vi "串口指令.vi"(7 "write buffer":string, 8 "error in":errorcluster, 9 "是否握手":bool=TRUE, 10 "limit":i32=200, 11 "VISA resource name":refnum<visa-resource-name>) -> (0 "error out":errorcluster, 1 "read buffer ALL":string, 2 "outputString":string, 3 "VISA resource name OUT":refnum<visa-resource-name>, 5 "read buffer HANDSHAKE":string)   [LabVIEW 2016]
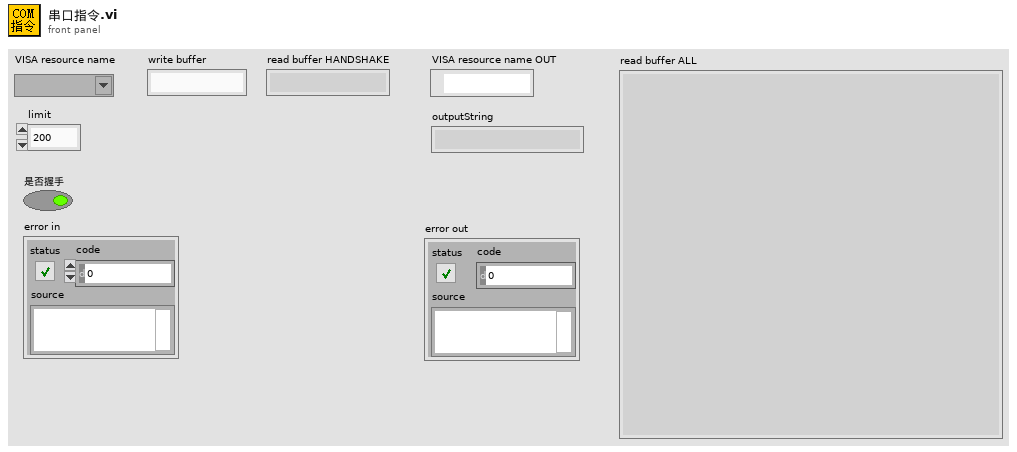
[diagram p1: front panel]
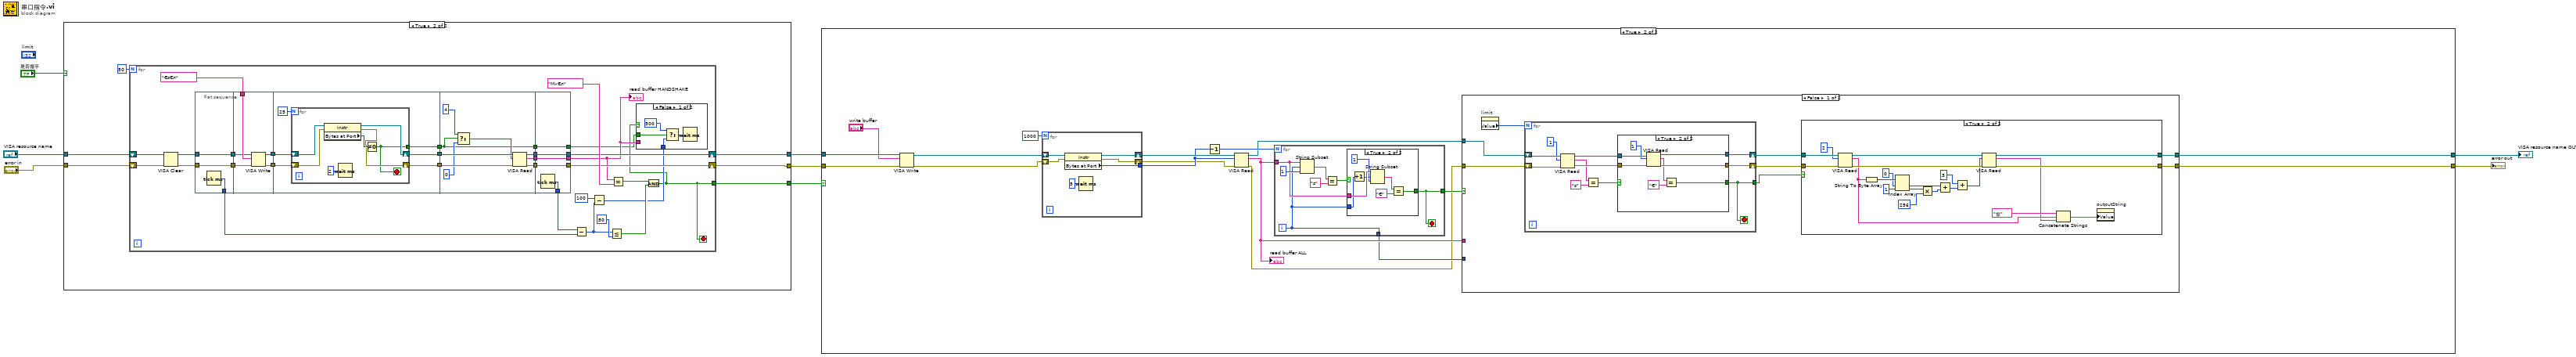
[diagram p0: block diagram]
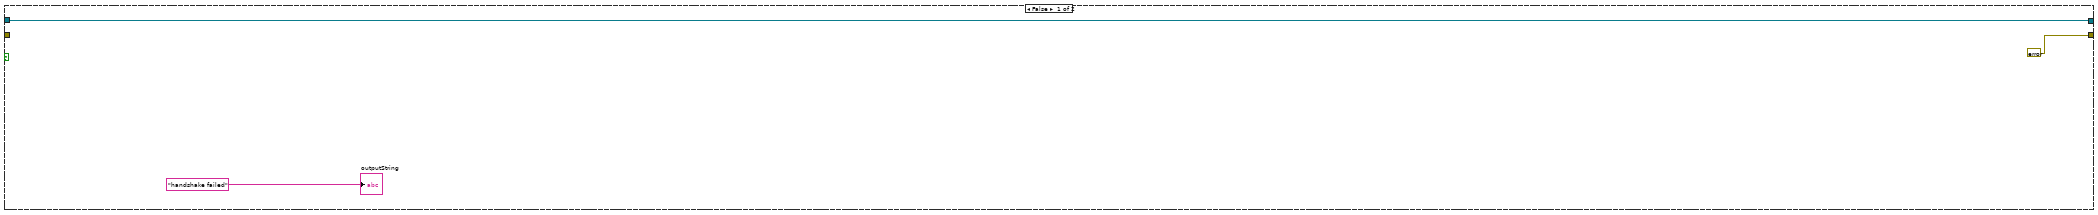
[diagram p2: hidden frame]
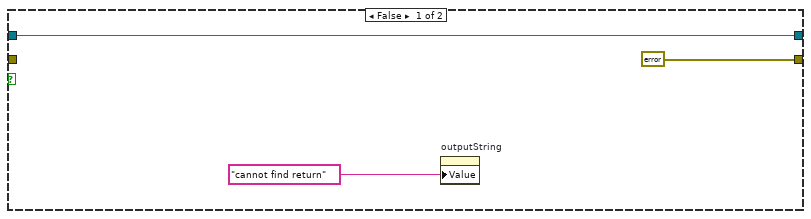
[diagram p3: hidden frame]
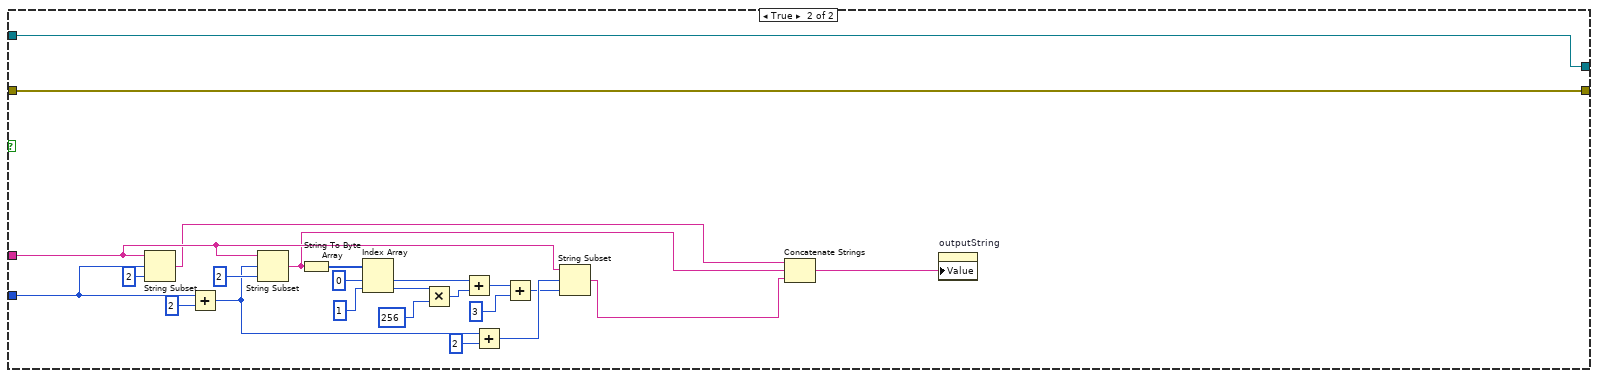
[diagram p5: hidden frame]
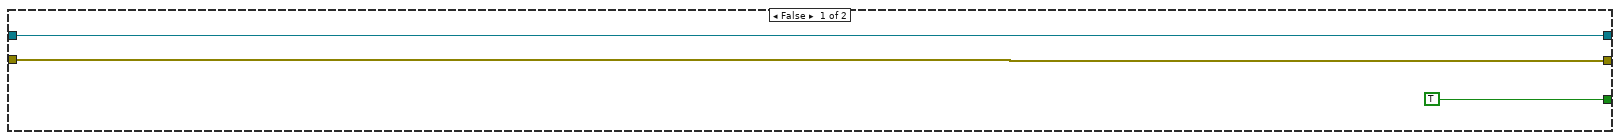
[diagram p7: hidden frame]
diagram:
  n1 = case shown="True" "是否握手" {
    tunnel: "VISA resource name" -> [w11 w16]
    tunnel: "error in" -> [w10 w15]
    tunnel: [w11 w13] -> w6
    tunnel: [w10 w12] -> w5
    tunnel: [TRUE w14] -> w4
    frame False {
    }
    frame True {
      n2 = for {
        N: 50 -> [_]
        shift-right: [w37] -> w13
        shift-left: w16 -> [w47]
        shift-right: [w35] -> w12
        shift-left: w15 -> [w44]
        tunnel: [w19] -> w14
        stop <- w19 stop-if-true
        n3 = VISA Clear(VISA resource name=w47, error in (no error)=w44) -> (VISA resource name out=w45:refnum<visa-resource-name>, error out=w43:errorcluster)
        n4 = flat-sequence {
          tunnel: [w54] -> w40
          tunnel: [w53] -> w39
          tunnel: [w52] -> w33
          tunnel: w45 -> [w54]
          tunnel: w43 -> [w53]
          tunnel: "ЄѕЄл" ("write buffer") -> [w59]
          tunnel: [w58] -> w29
          tunnel: [w57] -> w27
          tunnel: w40 -> [w56]
          tunnel: w39 -> [w55]
          tunnel: w29 -> [w65]
          tunnel: [w62] -> w28
          tunnel: w27 -> [w64]
          tunnel: [w61] -> w26
          tunnel: [w60] -> w25
          tunnel: w28 -> [w80]
          tunnel: w26 -> [w81]
          tunnel: [w79] -> w41
          tunnel: [w78] -> w38
          tunnel: [w77] -> w36
          tunnel: w25 -> [w73]
          tunnel: [w73] -> w24
          tunnel: [w86] -> w23
          tunnel: w41 -> [w86]
          tunnel: [w85] -> w34
          tunnel: [w84] -> w37
          tunnel: w38 -> [w84]
          tunnel: w36 -> [w83]
          tunnel: [w83] -> w35
          tunnel: w24 -> [w82]
          tunnel: [w82] -> w18
          frame #0 {
            n5 = Tick Count (ms)() -> (millisecond timer value=w52:u32)
          }
          frame #1 {
            n6 = VISA Write(VISA resource name=w56, write buffer=w59, error in (no error)=w55) -> (VISA resource name out=w58:refnum<visa-resource-name>, error out=w57:errorcluster)  [unwired: 1 out]
          }
          frame #2 {
            n7 = for {
              N: 25 -> [_]
              shift-right: [w69] -> w62
              shift-left: w65 -> [w72]
              shift-right: [w68] -> w61
              shift-left: w64 -> [w71]
              tunnel: [w66] -> w60
              stop <- w66 stop-if-true
              n8 = property class="Instr"(reference=w72, error in=w71) -> (reference out=w69:refnum<visa-resource-name>, error out=w68:errorcluster, "Bytes at Port"=w70:u32)
              n9 = Wait (ms)(milliseconds to wait=u32 2) -> ()  [unwired: 1 out]
              n10 = Not Equal To 0?(x=w70) -> (x != 0?=w66:bool)
            }
          }
          frame #3 {
            n11 = Select(t=u32 4 ("byte count"), s=w73, f=u32 0) -> (s? t:f=w74:u32)
            n12 = VISA Read(VISA resource name=w80, byte count=w74, error in (no error)=w81) -> (VISA resource name out=w78:refnum<visa-resource-name>, read buffer=w79:string, error out=w77:errorcluster)  [unwired: 1 out]
          }
          frame #4 {
            n13 = Tick Count (ms)() -> (millisecond timer value=w85:u32)
          }
        }
        n14 = Subtract(x=w34, y=w33) -> (x-y=w22:u32)
        n15 = Subtract(x=u32 100, y=w22) -> (x-y=w20:u32)
        n16 = Less Or Equal?(x=w22, y=u32 50) -> (x <= y?=w30:bool)
        n17 = Equal?(x=w23, y="М»Єл" ("write buffer")) -> (x = y?=w31:bool)
        n18 = And(x=w31, y=w30) -> (x .and. y?=w19:bool)
        n19 = case shown="False" w19 {
          tunnel: w23 -> [_ _]
          tunnel: w18 -> [w51 _]
          tunnel: w20 -> [w48 _]
          frame False {
            n20 = Select(t=u32 500 ("milliseconds to wait"), s=w51, f=w48) -> (s? t:f=w49:u32)
            n21 = Wait (ms)(milliseconds to wait=w49) -> ()  [unwired: 1 out]
          }
          frame True {
          }
        }
        "read buffer HANDSHAKE" <- w23
      }
    }
  }
  n22 = case shown="True" w4 {
    tunnel: w6 -> [w89 w106]
    tunnel: w5 -> [_ w105]
    tunnel: [w89 w104] -> w3
    tunnel: [errorcluster {"status"=TRUE, "code"=1000001, "source"="handshake failed"} ("error in") w103] -> w2
    frame False {
      "outputString" <- "handshake failed" ("string")
    }
    frame True {
      n23 = VISA Write(VISA resource name=w106, write buffer="write buffer", error in (no error)=w105) -> (VISA resource name out=w102:refnum<visa-resource-name>, error out=w100:errorcluster)  [unwired: 1 out]
      n24 = for {
        N: 1000 -> [_]
        shift-right: [w204] -> w99
        shift-left: w102 -> [w205]
        tunnel: [w203] -> w98
        shift-right: [w200] -> w94
        shift-left: w100 -> [w201]
        n25 = property class="Instr"(reference=w205, error in=w201) -> (reference out=w204:refnum<visa-resource-name>, error out=w200:errorcluster, "Bytes at Port"=w203:u32)
        n26 = Wait (ms)(milliseconds to wait=u32 5) -> ()  [unwired: 1 out]
      }
      n27 = Decrement(x=w98) -> (x-1=w97:u32)
      n28 = VISA Read(VISA resource name=w99, byte count=w98, error in (no error)=w94) -> (VISA resource name out=w95:refnum<visa-resource-name>, read buffer=w93:string, error out=w91:errorcluster)  [unwired: 1 out]
      "read buffer ALL" <- w93
      n29 = for {
        N: w97 -> [_]
        tunnel: w93 -> [w187]
        tunnel: [w186] -> w96
        tunnel: [w185] -> w92
        i -> [w185]
        stop <- w186 stop-if-true
        n30 = String Subset(string=w187, offset (0)=w185, length (rest)=1 ("length (rest)")) -> (substring=w190:string)
        n31 = Equal?(x=w190, y="ѕ") -> (x = y?=w188:bool)
        n32 = case shown="True" w188 {
          selector: w188 -> [w192 _]
          tunnel: w187 -> [_ w199]
          tunnel: w185 -> [_ w198]
          tunnel: [w192 w193] -> w186
          frame False {
          }
          frame True {
            n33 = Increment(x=w198) -> (x+1=w197:i32)
            n34 = String Subset(string=w199, offset (0)=w197, length (rest)=1 ("length (rest)")) -> (substring=w195:string)
            n35 = Equal?(x=w195, y="Є") -> (x = y?=w193:bool)
          }
        }
      }
      n36 = case shown="False" w96 {
        tunnel: [w112 w184] -> w104
        tunnel: [w111 w183] -> w103
        tunnel: w95 -> [w109 w184]
        tunnel: w91 -> [w108 w183]
        tunnel: w93 -> [_ w165]
        tunnel: w92 -> [_ w181]
        frame False {
          n37 = property on="limit" class="DigNum (strict)"() -> ("Value"=w107:i32)  [unwired: 2 in, 2 out]
          n38 = for {
            N: w107 -> [_]
            shift-right: [w142] -> w114
            shift-left: w109 -> [w149]
            shift-right: [w141] -> w113
            shift-left: w108 -> [w148]
            tunnel: [w140] -> w110
            stop <- w140 stop-if-true
            n39 = VISA Read(VISA resource name=w149, byte count=u32 1, error in (no error)=w148) -> (VISA resource name out=w144:refnum<visa-resource-name>, read buffer=w139:string, error out=w143:errorcluster)  [unwired: 1 out]
            n40 = Equal?(x=w139, y="ѕ") -> (x = y?=w145:bool)
            n41 = case shown="True" w145 {
              selector: w145 -> [w151 _]
              tunnel: w144 -> [w152 w160]
              tunnel: w143 -> [w150 w159]
              tunnel: [w152 w157] -> w142
              tunnel: [w150 w156] -> w141
              tunnel: [w151 w153] -> w140
              frame False {
              }
              frame True {
                n42 = VISA Read(VISA resource name=w160, byte count=u32 1, error in (no error)=w159) -> (VISA resource name out=w157:refnum<visa-resource-name>, read buffer=w155:string, error out=w156:errorcluster)  [unwired: 1 out]
                n43 = Equal?(x=w155, y="Є") -> (x = y?=w153:bool)
              }
            }
          }
          n44 = case shown="True" w110 {
            tunnel: w114 -> [w117 w137]
            tunnel: w113 -> [_ w138]
            tunnel: [errorcluster {"status"=TRUE, "code"=1000002, "source"="cannot find return"} ("error out") w135] -> w111
            tunnel: [w117 w134] -> w112
            frame False {
              n45 = property on="outputString" class="Str"("Value"="cannot find return" ("string")) -> ()  [unwired: 2 in, 2 out]
            }
            frame True {
              n46 = VISA Read(VISA resource name=w137, byte count=u32 2, error in (no error)=w138) -> (VISA resource name out=w124:refnum<visa-resource-name>, read buffer=w119:string, error out=w125:errorcluster)  [unwired: 1 out]
              n47 = String To Byte Array(string=w119) -> (unsigned byte array=w132:u8[])
              n48 = Index Array(array=w132, index #1=0 ("index"), index #2=1 ("index")) -> (element #1=w126:u8, element #2=w128:u8)
              n49 = Multiply(x=w128, y=u16 256) -> (x*y=w127:u16)
              n50 = Add(x=w126, y=w127) -> (x+y=w123:u16)
              n51 = Add(x=u16 3, y=w123) -> (x+y=w122:u16)
              n52 = VISA Read(VISA resource name=w124, byte count=w122, error in (no error)=w125) -> (VISA resource name out=w134:refnum<visa-resource-name>, read buffer=w118:string, error out=w135:errorcluster)  [unwired: 1 out]
              n53 = Concatenate Strings("惊" ("String"), w119, w118) -> (w136:string)
              n54 = property on="outputString" class="Str"("Value"=w136) -> ()  [unwired: 2 in, 2 out]
            }
          }
        }
        frame True {
          n55 = String Subset(string=w165, offset (0)=w181, length (rest)=2 ("length (rest)")) -> (substring=w164:string)
          n56 = Add(x=w181, y=2) -> (x+y=w171:i32)
          n57 = String Subset(string=w165, offset (0)=w171, length (rest)=2 ("length (rest)")) -> (substring=w163:string)
          n58 = String To Byte Array(string=w163) -> (unsigned byte array=w178:u8[])
          n59 = Index Array(array=w178, index #1=0 ("index"), index #2=1 ("index")) -> (element #1=w172:u8, element #2=w175:u8)
          n60 = Multiply(x=w175, y=u16 256) -> (x*y=w173:u16)
          n61 = Add(x=w172, y=w173) -> (x+y=w168:u16)
          n62 = Add(x=w171, y=2) -> (x+y=w169:i32)
          n63 = Add(x=w168, y=u16 3) -> (x+y=w167:u16)
          n64 = String Subset(string=w165, offset (0)=w169, length (rest)=w167) -> (substring=w162:string)
          n65 = Concatenate Strings(w164, w163, w162) -> (w161:string)
          n66 = property on="outputString" class="Str"("Value"=w161) -> ()  [unwired: 2 in, 2 out]
        }
      }
    }
  }
  "VISA resource name OUT" <- w3
  "error out" <- w2
